vi "ExperimentStateLoad.vi"(4 "Previous Shot #":i32, 5 "Current ExpState IN":T1={"error"={"status"=FALSE, "code"=0, "source"=""}, "Digitizer DAQmx Tasks"={"TaskArray"=[]}, "DAQ Settings"={"Channel Settings"=[], "Card Settings"=[]}, "Synchronization Settings"={"Synchronizer 0"="PXI1Slot2", "source terminal"="GlobalSoftwareTrigger", "Synchronizer 1"="PXI1Slot2"}, "DAQ Data"=[], "Next Shot#"="0", "System Message"="", "User Shot Notes"="", "Timing Settings"={"Timing Card Settings"=[], "Timing Channel Settings"=[[{"Delay (s)"=2.559999942779541, "Pulse width (s)"=0.009999999776482582, "Active"=TRUE, "Channel Name"="Fiber 8", "counter"="PXI1Slot8/ctr7", "FrontPanelTime"=2.559999942779541}]]}, "Timing Tasks"={"TaskArray"=[]}, "Tree"="0", "Time Card/Channels"=[2, 8], "DAQ Card/Channels"=[3, 8], "Program Version"="", "RIO Settings"={"Channel Settings"=[], "Card Settings"=[]}, "RIO References"={"Reference Array"=[]}, "RIO Data"={"RIO Deleaved Data"=[], "Raw Readout"=[]}, "RIO Card/Channels"=[3, 8], "DIO Channels"=0, "DIO Settings"={"DIO Channel Array"=[]}, "Global Settings"={"Initial Background Values"={"Reference Shot #"=0.0, "Background pressure [Torr]"=0.0, "Cryo temp [V]"=0.0, "Cryo temp [K]"=0.0, "Cryotemp Calibration File"=path ""}, "Gas Puffing"={"Gas A type"="N", "Gas B type"="N", "Gas C type"="N", "Gas A pressure [psi]"=0.0, "Gas B pressure [psi]"=0.0, "Gas C pressure [psi]"=0.0, "Innner Electrode"="", "Middle Electrode"="", "Outer Electrode"="", "Gas A bottle pressure [psi]"=0.0, "Gas B bottle pressure [psi]"=0.0, "Gas C bottle pressure [psi]"=0.0}, "PSU Voltages"={"Bias1 Voltage [V]"=0.0, "Bias2 Voltage [V]"=0.0, "PSU1 Voltage [V]"=0.0, "Puff-PSU1 CH1 Voltage [V]"=0.0, "Puff-PSU1 CH2 Voltage [V]"=0.0, "Puff-PSU1 CH3 Voltage [V]"=0.0, "PSU2 Voltage [V]"=0.0, "PSU3 Voltage [V]"=0.0}, "TEK 2024B - TEK - Details"={"CH1"="", "CH2"="", "CH3"="", "CH4"="", "CH1 Ground State"="Grounded", "CH2 Ground State"="Grounded", "CH3 Ground State"="Grounded", "CH4 Ground State"="Grounded"}, "TEK 2024B - TEK1 - Details"={"CH1"="", "CH2"="", "CH3"="", "CH4"="", "CH1 Ground State"="Grounded", "CH2 Ground State"="Grounded", "CH3 Ground State"="Grounded", "CH4 Ground State"="Grounded"}}, "Calibrations"={"CryoTemp"={"Comment"="", "X"=[], "Y"=[]}, "PSU2 Tach"={"Comment"="", "X"=[], "Y"=[]}, "PSU3 Tach"={"Comment"="", "X"=[], "Y"=[]}, "PSU2 RevTach"={"Comment"="", "X"=[], "Y"=[]}, "PSU3 RevTach"={"Comment"="", "X"=[], "Y"=[]}}, "Tach Tasks"={"PSU2 task"="", "PSU3 task"=""}, "PSU2 Panel Settings"={"PSU2 DIO channels"={"Charge relay DIO"="DAQ0/port0/line3", "Dump relay DIO"="DAQ0/port0/line4", "HV Arm DIO"="DAQ0/port0/line5", "HV On DIO"="DAQ0/port0/line6"}, "PSU2 Tachometer Controls"={"PSU2 Tach Calibration"=path "Z:/Data/Calibration/Tachometer", "PSU2 Charging Voltage [kV]"=0.0, "PSU2 Tach Counter"="DAQ0/port0/line3"}, "PSU2 Reverse Tachometer Controls"={"PSU2 RevTach Calibration"=path "Z:/Data/Calibration/Reverse Tachometer/PSU2_RevTachCalibration.csv", "PSU2 bank Voltage [kV]"=0.0, "PSU2 RevTach Counter"=""}}, "PSU3 Panel Settings"={"PSU3 DIO channels"={"Charge relay DIO"="DAQ0/port0/line5", "Dump relay DIO"="DAQ0/port0/line6", "HV Arm DIO"="", "HV On DIO"="DAQ0/port0/line6"}, "PSU3 Tachometer Controls"={"PSU3 Tach Calibration"=path "Z:/Data/Calibration/Reverse Tachometer/PSU3_RevTachCalibration.csv", "PSU3 Charging Voltage [kV]"=0.0, "PSU3 Tach Counter"=""}, "PSU3 Reverse Tachometer Controls"={"PSU3 RevTach Calibration"=path "Z:/Data/Calibration/Reverse Tachometer/PSU3_RevTachCalibration.csv", "PSU3 bank Voltage [kV]"=0.0, "PSU3 RevTach Counter"=""}}} {"Global Settings"."Initial Background Values"."Cryo temp [K]" format="%#_4g"; "RIO Settings"."Card Settings"."Digital High \nPass Filter k" items=["10"=21, "9"=19, "8"=17, "7"=15, "6"=13, "5"=11, "4"=9, "3"=7, "2"=5, "Off"=0]; "RIO Settings"."Card Settings"."Sample Rate" format="%#_3p"; "Timing Settings"."Timing Channel Settings"."FrontPanelTime" format="%.3p"; "Timing Settings"."Timing Channel Settings"."Pulse width (s)" format="%.3p"; "Timing Settings"."Timing Channel Settings"."Delay (s)" format="%.3p"; "DAQ Settings"."Card Settings"."Global Edge Type" items=["Rising"=10280, "Falling"=10171]; "DAQ Settings"."Card Settings"."Sample Rate" format="%#_3p"}) -> (0 "Error out":errorcluster, 1 "Updated ExpState OUT":T1={"error"={"status"=FALSE, "code"=0, "source"=""}, "Digitizer DAQmx Tasks"={"TaskArray"=[]}, "DAQ Settings"={"Channel Settings"=[], "Card Settings"=[]}, "Synchronization Settings"={"Synchronizer 0"="PXI1Slot2", "source terminal"="GlobalSoftwareTrigger", "Synchronizer 1"="PXI1Slot2"}, "DAQ Data"=[], "Next Shot#"="0", "System Message"="", "User Shot Notes"="", "Timing Settings"={"Timing Card Settings"=[], "Timing Channel Settings"=[[{"Delay (s)"=2.559999942779541, "Pulse width (s)"=0.009999999776482582, "Active"=TRUE, "Channel Name"="Fiber 8", "counter"="PXI1Slot8/ctr7", "FrontPanelTime"=2.559999942779541}]]}, "Timing Tasks"={"TaskArray"=[]}, "Tree"="0", "Time Card/Channels"=[2, 8], "DAQ Card/Channels"=[3, 8], "Program Version"="", "RIO Settings"={"Channel Settings"=[], "Card Settings"=[]}, "RIO References"={"Reference Array"=[]}, "RIO Data"={"RIO Deleaved Data"=[], "Raw Readout"=[]}, "RIO Card/Channels"=[3, 8], "DIO Channels"=0, "DIO Settings"={"DIO Channel Array"=[]}, "Global Settings"={"Initial Background Values"={"Reference Shot #"=0.0, "Background pressure [Torr]"=0.0, "Cryo temp [V]"=0.0, "Cryo temp [K]"=0.0, "Cryotemp Calibration File"=path ""}, "Gas Puffing"={"Gas A type"="N", "Gas B type"="N", "Gas C type"="N", "Gas A pressure [psi]"=0.0, "Gas B pressure [psi]"=0.0, "Gas C pressure [psi]"=0.0, "Innner Electrode"="", "Middle Electrode"="", "Outer Electrode"="", "Gas A bottle pressure [psi]"=0.0, "Gas B bottle pressure [psi]"=0.0, "Gas C bottle pressure [psi]"=0.0}, "PSU Voltages"={"Bias1 Voltage [V]"=0.0, "Bias2 Voltage [V]"=0.0, "PSU1 Voltage [V]"=0.0, "Puff-PSU1 CH1 Voltage [V]"=0.0, "Puff-PSU1 CH2 Voltage [V]"=0.0, "Puff-PSU1 CH3 Voltage [V]"=0.0, "PSU2 Voltage [V]"=0.0, "PSU3 Voltage [V]"=0.0}, "TEK 2024B - TEK - Details"={"CH1"="", "CH2"="", "CH3"="", "CH4"="", "CH1 Ground State"="Grounded", "CH2 Ground State"="Grounded", "CH3 Ground State"="Grounded", "CH4 Ground State"="Grounded"}, "TEK 2024B - TEK1 - Details"={"CH1"="", "CH2"="", "CH3"="", "CH4"="", "CH1 Ground State"="Grounded", "CH2 Ground State"="Grounded", "CH3 Ground State"="Grounded", "CH4 Ground State"="Grounded"}}, "Calibrations"={"CryoTemp"={"Comment"="", "X"=[], "Y"=[]}, "PSU2 Tach"={"Comment"="", "X"=[], "Y"=[]}, "PSU3 Tach"={"Comment"="", "X"=[], "Y"=[]}, "PSU2 RevTach"={"Comment"="", "X"=[], "Y"=[]}, "PSU3 RevTach"={"Comment"="", "X"=[], "Y"=[]}}, "Tach Tasks"={"PSU2 task"="", "PSU3 task"=""}, "PSU2 Panel Settings"={"PSU2 DIO channels"={"Charge relay DIO"="DAQ0/port0/line3", "Dump relay DIO"="DAQ0/port0/line4", "HV Arm DIO"="DAQ0/port0/line5", "HV On DIO"="DAQ0/port0/line6"}, "PSU2 Tachometer Controls"={"PSU2 Tach Calibration"=path "Z:/Data/Calibration/Tachometer", "PSU2 Charging Voltage [kV]"=0.0, "PSU2 Tach Counter"="DAQ0/port0/line3"}, "PSU2 Reverse Tachometer Controls"={"PSU2 RevTach Calibration"=path "Z:/Data/Calibration/Reverse Tachometer/PSU2_RevTachCalibration.csv", "PSU2 bank Voltage [kV]"=0.0, "PSU2 RevTach Counter"=""}}, "PSU3 Panel Settings"={"PSU3 DIO channels"={"Charge relay DIO"="DAQ0/port0/line5", "Dump relay DIO"="DAQ0/port0/line6", "HV Arm DIO"="", "HV On DIO"="DAQ0/port0/line6"}, "PSU3 Tachometer Controls"={"PSU3 Tach Calibration"=path "Z:/Data/Calibration/Reverse Tachometer/PSU3_RevTachCalibration.csv", "PSU3 Charging Voltage [kV]"=0.0, "PSU3 Tach Counter"=""}, "PSU3 Reverse Tachometer Controls"={"PSU3 RevTach Calibration"=path "Z:/Data/Calibration/Reverse Tachometer/PSU3_RevTachCalibration.csv", "PSU3 bank Voltage [kV]"=0.0, "PSU3 RevTach Counter"=""}}} {"Global Settings"."Initial Background Values"."Cryo temp [K]" format="%#_4g"; "RIO Settings"."Card Settings"."Digital High \nPass Filter k" items=["10"=21, "9"=19, "8"=17, "7"=15, "6"=13, "5"=11, "4"=9, "3"=7, "2"=5, "Off"=0]; "RIO Settings"."Card Settings"."Sample Rate" format="%#_3p"; "Timing Settings"."Timing Channel Settings"."FrontPanelTime" format="%.3p"; "Timing Settings"."Timing Channel Settings"."Pulse width (s)" format="%.3p"; "Timing Settings"."Timing Channel Settings"."Delay (s)" format="%.3p"; "DAQ Settings"."Card Settings"."Global Edge Type" items=["Rising"=10280, "Falling"=10171]; "DAQ Settings"."Card Settings"."Sample Rate" format="%#_3p"})   [LabVIEW 2015]
uses:
  Controls/ExperimentStateCluster.ctl
  Controls/DigitizerSettingsChannelSettings.ctl
  Controls/DigitizerSettingsCardSettingsArray.ctl
  Controls/DigitizerSettingsCardSettings.ctl
  Controls/TimingSettings.ctl
  Controls/TimingCardSettings.ctl
  Controls/TimingChannelSettings.ctl
  Controls/RIOSettingsExperimentStateCluster.ctl
  Controls/RIOChannelSettingsArrayExperimentStateCluster.ctl
  Controls/RIOSettingsChannelSettings.ctl
  Controls/RIOSettingsCardSettingsArray.ctl
  Controls/RIOSettingsCardSettings.ctl
  <vilib>/userdefined/High Color/nirio_resource_hc.ctl
  Controls/DigitalHighPassFilter.ctl
  Controls/RIOData.ctl
  Controls/DIOChannel.ctl
  Controls/Global Settings/GlobalSettings.ctl
  Controls/Global Settings/InitialBackgroundValues.ctl
  Controls/Global Settings/GasPuffing.ctl
  Controls/Global Settings/PSUVoltages.ctl
  Controls/Global Settings/ScopeDetails.ctl
  Controls/Calibrations/Calibrations.ctl
  Controls/Calibrations/CryoTemoCalibration.ctl
  Controls/Calibrations/PSU2TachCalibration.ctl
  Controls/Calibrations/PSU3TachCalibration.ctl
  Controls/TachTasks.ctl
  Controls/PSU2PanelSettings.ctl
  Controls/PSU2DIOChannels.ctl
  Controls/PSU2TachometerControls.ctl
  Controls/PSU2ReverseTachometerControls.ctl
  Controls/PSU3PanelSettings.ctl
  Controls/PSU3DIOChannels.ctl
  Controls/PSU3TachometerControls.ctl
  Controls/PSU3ReverseTachometerControls.ctl
  <vilib>/MDSplus/Library/MDSplus.lvlib
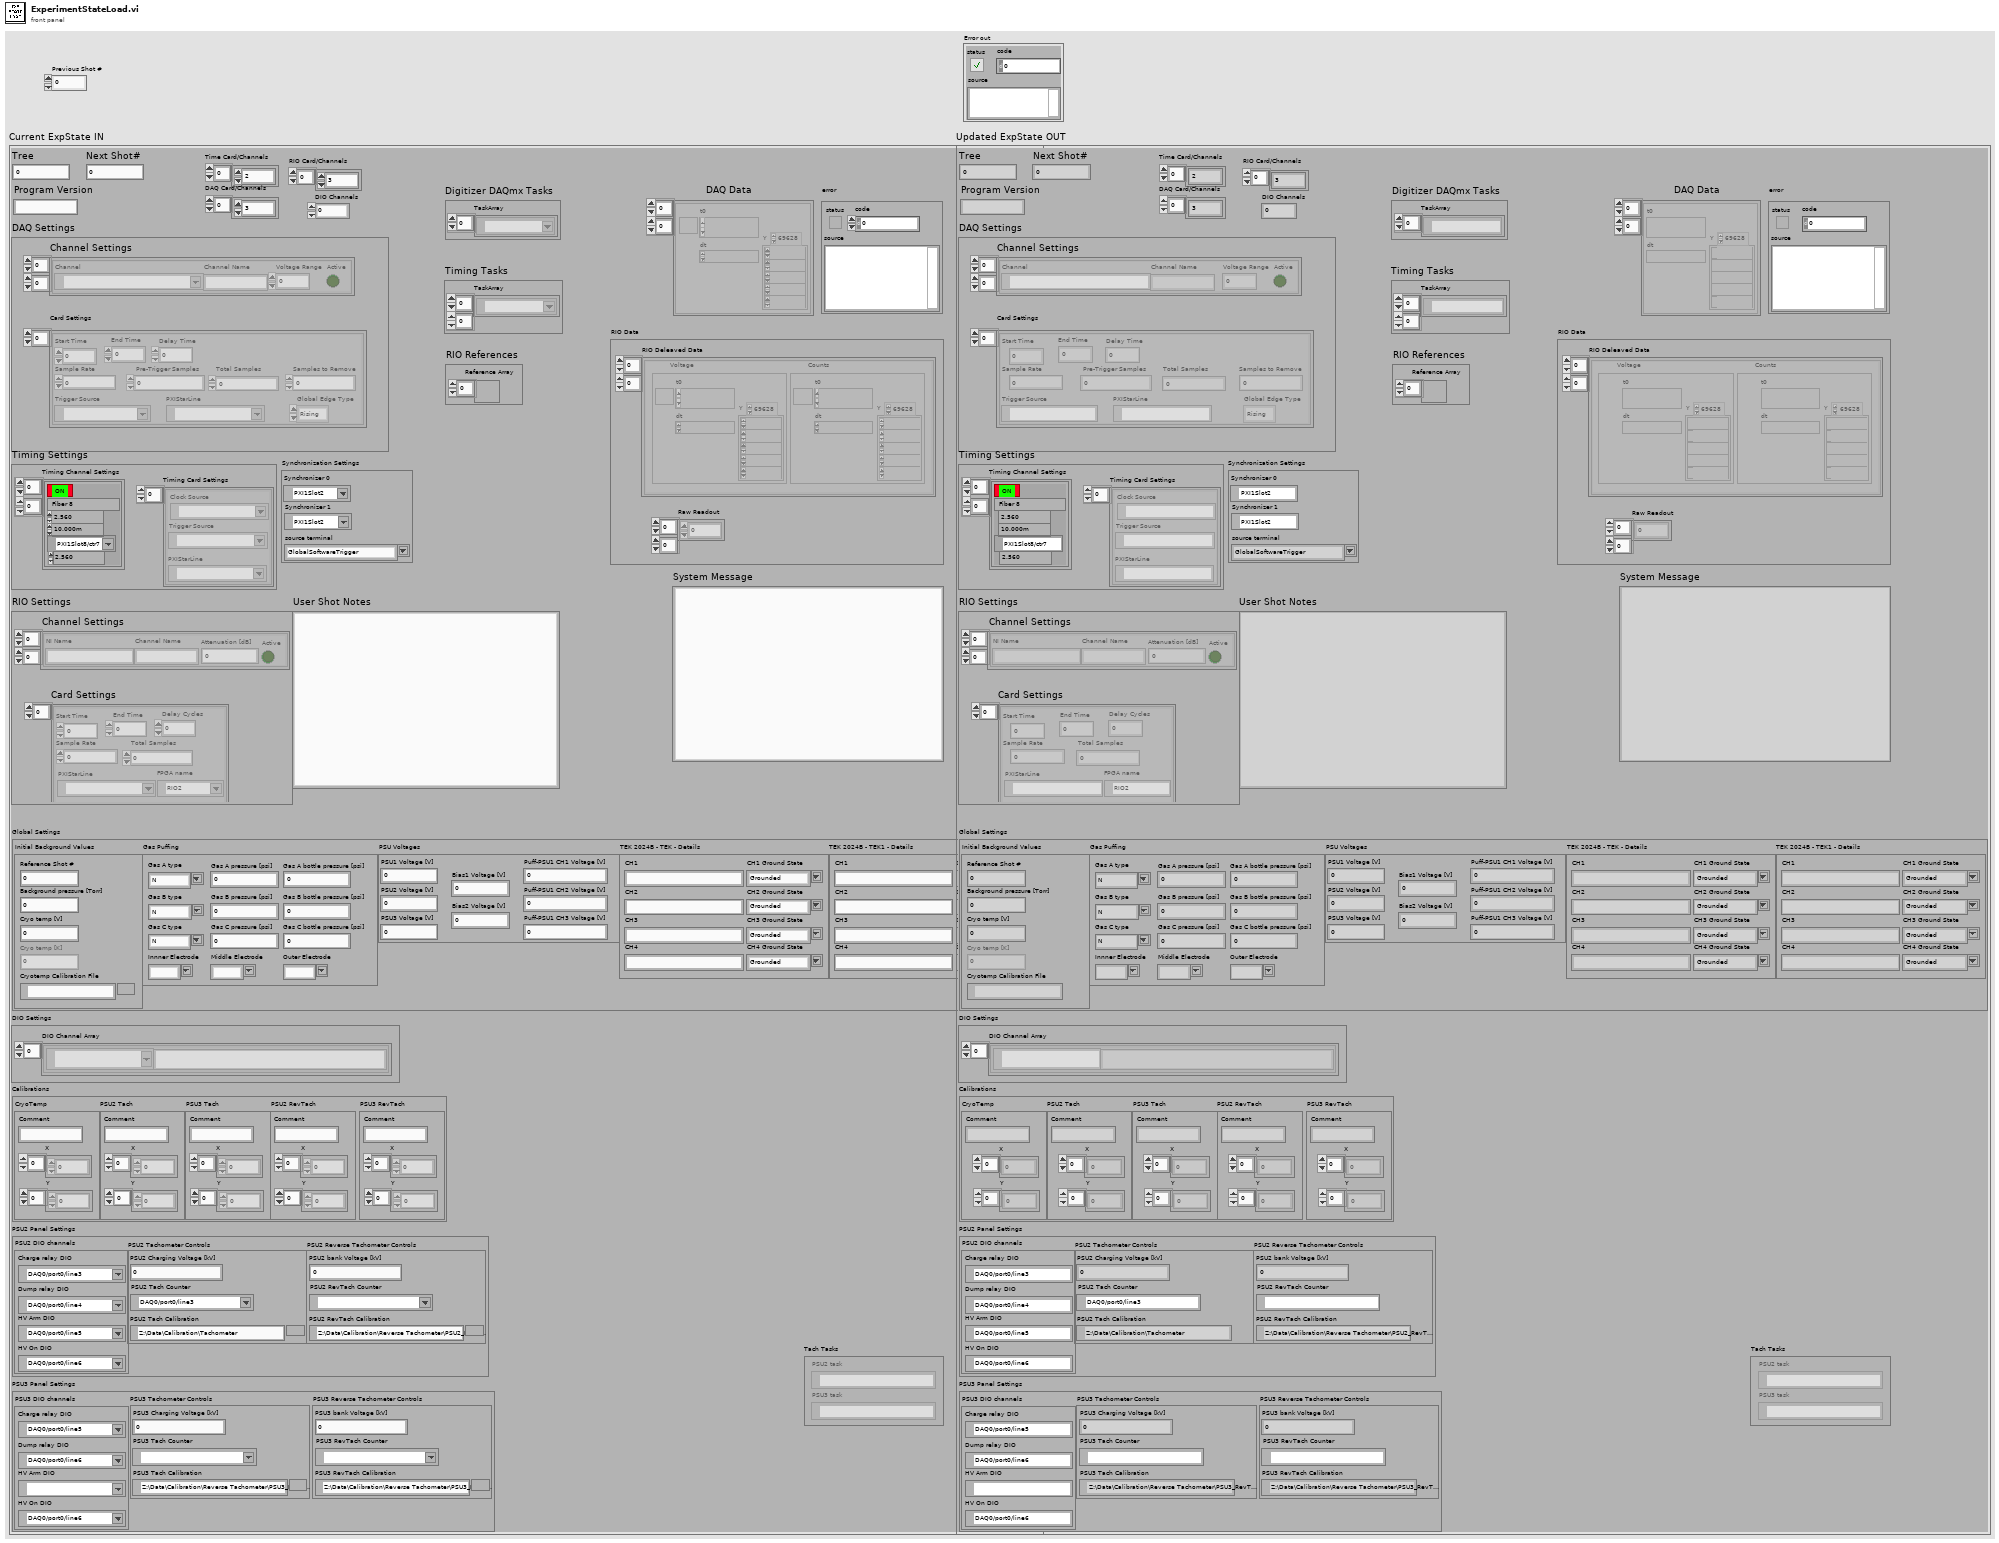
[diagram p1: front panel]
types:
  T1 = typedef "ExperimentStateCluster.ctl" = cluster{"error":errorcluster, "Digitizer DAQmx Tasks":cluster{"TaskArray":refnum<k21>[]}, "DAQ Settings":cluster{"Channel Settings":T2[][], "Card Settings":T3}, "Synchronization Settings":cluster{"Synchronizer 0":refnum<k15>, "source terminal":string, "Synchronizer 1":refnum<k15>}, "DAQ Data":waveform(dbl)[][], "Next Shot#":string, "System Message":string, "User Shot Notes":string, "Timing Settings":T5, "Timing Tasks":cluster{"TaskArray":refnum<k21>[][]}, "Tree":string, "Time Card/Channels":i32[], "DAQ Card/Channels":i32[], "Program Version":string, "RIO Settings":T8, "RIO References":cluster{"Reference Array":refnum<k20>[]}, "RIO Data":T15, "RIO Card/Channels":i32[], "DIO Channels":i32, "DIO Settings":cluster{"DIO Channel Array":T16[]}, "Global Settings":T17, "Calibrations":T22, "Tach Tasks":T26, "PSU2 Panel Settings":T27, "PSU3 Panel Settings":T31}
  T2 = typedef "DigitizerSettingsChannelSettings.ctl" = cluster{"Channel":tag, "Channel Name":string, "Voltage Range":dbl, "Active":bool}
  T3 = typedef "DigitizerSettingsCardSettingsArray.ctl" = T4[]
  T4 = typedef "DigitizerSettingsCardSettings.ctl" = cluster{"Start Time":dbl, "End Time":dbl, "Sample Rate":dbl, " Pre-Trigger Samples":u32, "Total Samples":i32, "Samples to Remove":u32, "Trigger Source":tag, "Global Edge Type":i32, "PXIStarLine":tag, "Delay Time":dbl}
  T5 = typedef "TimingSettings.ctl" = cluster{"Timing Card Settings":T6[], "Timing Channel Settings":T7[][]}
  T6 = typedef "TimingCardSettings.ctl" = cluster{"Trigger Source":tag, "Clock Source":tag, "PXIStarLine":tag}
  T7 = typedef "TimingChannelSettings.ctl" = cluster{"Delay (s)":dbl, "Pulse width (s)":dbl, "Active":bool, "Channel Name":string, "counter":tag, "FrontPanelTime":dbl}
  T8 = typedef "RIOSettingsExperimentStateCluster.ctl" = cluster{"Channel Settings":T9, "Card Settings":T11}
  T9 = typedef "RIOChannelSettingsArrayExperimentStateCluster.ctl" = T10[][]
  T10 = typedef "RIOSettingsChannelSettings.ctl" = cluster{"Channel Name":string, "Active":bool, "NI Name":string, "Attenuation [dB]":i32}
  T11 = typedef "RIOSettingsCardSettingsArray.ctl" = T12[]
  T12 = typedef "RIOSettingsCardSettings.ctl" = cluster{"Start Time":dbl, "End Time":dbl, "Sample Rate":dbl, "Total Samples":u64, "PXIStarLine":tag, "Delay Cycles":u64, "FPGA name":T13, "Digital High \nPass Filter k":T14}
  T13 = typedef "nirio_resource_hc.ctl" = tag
  T14 = typedef "DigitalHighPassFilter.ctl" = u16
  T15 = typedef "RIOData.ctl" = cluster{"RIO Deleaved Data":cluster{"Voltage":waveform(dbl), "Counts":waveform(i16)}[][], "Raw Readout":u64[][]}
  T16 = typedef "DIOChannel.ctl" = cluster{"Channel Name":string, "NI Name":tag}
  T17 = typedef "GlobalSettings.ctl" = cluster{"Initial Background Values":T18, "Gas Puffing":T19, "PSU Voltages":T20, "TEK 2024B - TEK - Details":T21, "TEK 2024B - TEK1 - Details":T21}
  T18 = typedef "InitialBackgroundValues.ctl" = cluster{"Reference Shot #":dbl, "Background pressure [Torr]":dbl, "Cryo temp [V]":dbl, "Cryo temp [K]":dbl, "Cryotemp Calibration File":path}
  T19 = typedef "GasPuffing.ctl" = cluster{"Gas A type":string, "Gas B type":string, "Gas C type":string, "Gas A pressure [psi]":dbl, "Gas B pressure [psi]":dbl, "Gas C pressure [psi]":dbl, "Innner Electrode":string, "Middle Electrode":string, "Outer Electrode":string, "Gas A bottle pressure [psi]":dbl, "Gas B bottle pressure [psi]":dbl, "Gas C bottle pressure [psi]":dbl}
  T20 = typedef "PSUVoltages.ctl" = cluster{"Bias1 Voltage [V]":dbl, "Bias2 Voltage [V]":dbl, "PSU1 Voltage [V]":dbl, "Puff-PSU1 CH1 Voltage [V]":dbl, "Puff-PSU1 CH2 Voltage [V]":dbl, "Puff-PSU1 CH3 Voltage [V]":dbl, "PSU2 Voltage [V]":dbl, "PSU3 Voltage [V]":dbl}
  T21 = typedef "ScopeDetails.ctl" = cluster{"CH1":string, "CH2":string, "CH3":string, "CH4":string, "CH1 Ground State":string, "CH2 Ground State":string, "CH3 Ground State":string, "CH4 Ground State":string}
  T22 = typedef "Calibrations.ctl" = cluster{"CryoTemp":T23, "PSU2 Tach":T24, "PSU3 Tach":T25, "PSU2 RevTach":T24, "PSU3 RevTach":T25}
  T23 = typedef "CryoTemoCalibration.ctl" = cluster{"Comment":string, "X":dbl[], "Y":dbl[]}
  T24 = typedef "PSU2TachCalibration.ctl" = cluster{"Comment":string, "X":dbl[], "Y":dbl[]}
  T25 = typedef "PSU3TachCalibration.ctl" = cluster{"Comment":string, "X":dbl[], "Y":dbl[]}
  T26 = typedef "TachTasks.ctl" = cluster{"PSU2 task":refnum<k21>, "PSU3 task":refnum<k21>}
  T27 = typedef "PSU2PanelSettings.ctl" = cluster{"PSU2 DIO channels":T28, "PSU2 Tachometer Controls":T29, "PSU2 Reverse Tachometer Controls":T30}
  T28 = typedef "PSU2DIOChannels.ctl" = cluster{"Charge relay DIO":tag, "Dump relay DIO":tag, "HV Arm DIO":tag, "HV On DIO":tag}
  T29 = typedef "PSU2TachometerControls.ctl" = cluster{"PSU2 Tach Calibration":path, "PSU2 Charging Voltage [kV]":dbl, "PSU2 Tach Counter":tag}
  T30 = typedef "PSU2ReverseTachometerControls.ctl" = cluster{"PSU2 RevTach Calibration":path, "PSU2 bank Voltage [kV]":dbl, "PSU2 RevTach Counter":tag}
  T31 = typedef "PSU3PanelSettings.ctl" = cluster{"PSU3 DIO channels":T32, "PSU3 Tachometer Controls":T33, "PSU3 Reverse Tachometer Controls":T34}
  T32 = typedef "PSU3DIOChannels.ctl" = cluster{"Charge relay DIO":tag, "Dump relay DIO":tag, "HV Arm DIO":tag, "HV On DIO":tag}
  T33 = typedef "PSU3TachometerControls.ctl" = cluster{"PSU3 Tach Calibration":path, "PSU3 Charging Voltage [kV]":dbl, "PSU3 Tach Counter":tag}
  T34 = typedef "PSU3ReverseTachometerControls.ctl" = cluster{"PSU3 RevTach Calibration":path, "PSU3 bank Voltage [kV]":dbl, "PSU3 RevTach Counter":tag}
  T35 = cluster{"Channel Settings":T2[][], "Card Settings":T3}
  T36 = typedef "DIOSettingsExperimentStateCluster.ctl" = cluster{"DIO Channel Array":T16[]}
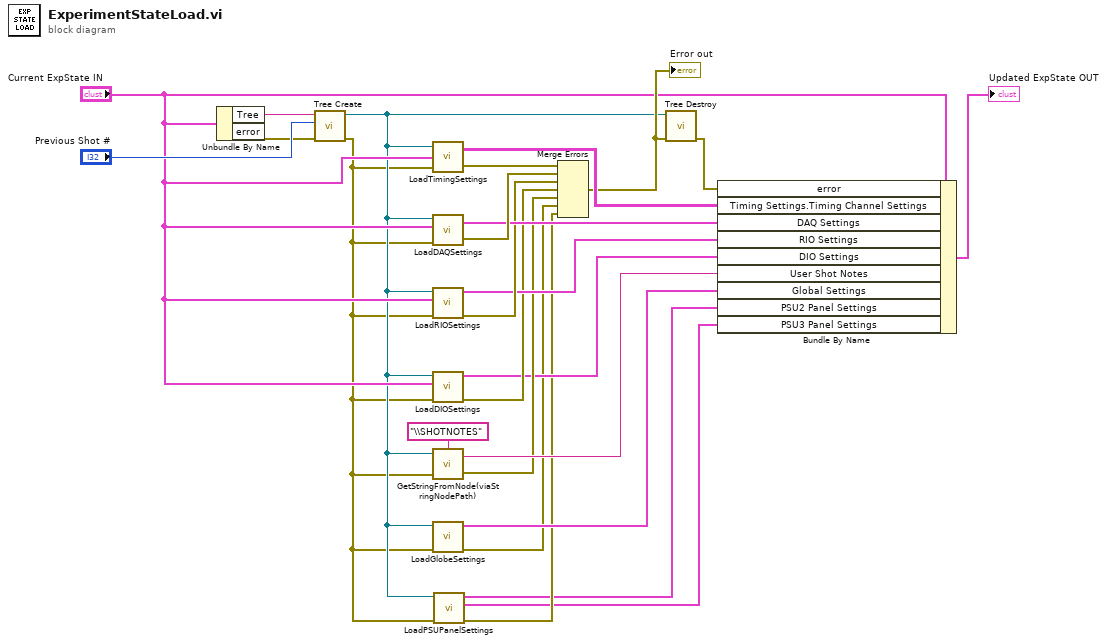
[diagram p0: block diagram]
diagram:
  n1 = Unbundle By Name("Current ExpState IN") -> ("Tree"=w18:string, "error"=w17:errorcluster)
  n2 = call <vilib>:"Tree Create.vi"("error in (no error)"=w17, "Shot"="Previous Shot #", "Name"=w18) -> ("error out"=w4:errorcluster, "Tree DVR out"=w5:refnum<data-value>)  [unwired: 7 in]
  n3 = call "LoadTimingSettings.vi"("error in (no error)"=w4, "Current ExpState IN"="Current ExpState IN", "Tree DVR In"=w5) -> ("error out"=w21:errorcluster, "Timing Card Settings"=w22:T7[][])
  n4 = call "LoadDAQSettings.vi"("error in"=w4, "Current ExpState IN"="Current ExpState IN", "Tree DVR In"=w5) -> ("error out"=w20:errorcluster, "Digitizer Settings"=w19:T35)  [unwired: 1 in]
  n5 = call "LoadRIOSettings.vi"("Error in"=w4, "Current ExpState IN"="Current ExpState IN", "Tree DVR in"=w5) -> ("Error out"=w14:errorcluster, "RIO Settings"=w12:T8)  [unwired: 7 in]
  n6 = call "LoadDIOSettings.vi"("Error in"=w4, "Current ExpState IN"="Current ExpState IN", "Tree DVR in"=w5) -> ("Error out"=w11:errorcluster, "DIO Settings"=w9:T36)  [unwired: 7 in]
  n7 = call "GetStringFromNode(viaStringNodePath).vi"("Path"="\\SHOTNOTES", "error in"=w4, "Tree DVR in"=w5) -> ("error out"=w10:errorcluster, "String out"=w13:string)  [unwired: 1 in]
  n8 = call "LoadGlobeSettings.vi"("error in (no error)"=w4, "Tree DVR in"=w5) -> ("error out"=w7:errorcluster, "Global Settings"=w8:T17)  [unwired: 8 in]
  n9 = call "LoadPSUPanelSettings.vi"("error in (no error)"=w4, "Tree DVR in"=w5) -> ("error out"=w3:errorcluster, "PSU3 Panel Settings"=w1:T31, "PSU2 Panel Settings"=w2:T27)  [unwired: 7 in]
  n10 = Merge Errors(w21, w20, w14, w11, w10, w7, w3) -> (w16:errorcluster)
  "Error out" <- w16
  n11 = call <vilib>:"Tree Destroy.vi"("error in (no error)"=w16, "Tree DVR in"=w5) -> ("error out"=w15:errorcluster)  [unwired: 9 in]
  n12 = Bundle By Name(cluster="Current ExpState IN", "error"=w15, "Timing Settings.Timing Channel Settings"=w22, "DAQ Settings"=w19, "RIO Settings"=w12, "DIO Settings"=w9, "User Shot Notes"=w13, "Global Settings"=w8, "PSU2 Panel Settings"=w2, "PSU3 Panel Settings"=w1) -> (→"Updated ExpState OUT":T1)
